vi "tapa color.vi"(9 "y":dbl=0.75, 10 "x":dbl=0.75, 11 "Image 2":T1) -> ()   [LabVIEW 2020]
uses:
  <vilib>/vision/Image Controls.llb/IMAQ Image.ctl
  <vilib>/vision/NI_Vision_Development_Module.lvlib
panel:
  out "Image":T1(plugin-control)
  in  "Color Sensitivity":u32(ring) items=["Low", "Medium", "High"]
  out "K":bool
  out "Color Spectrum":dbl[](array[numeric]) format="%.2f"
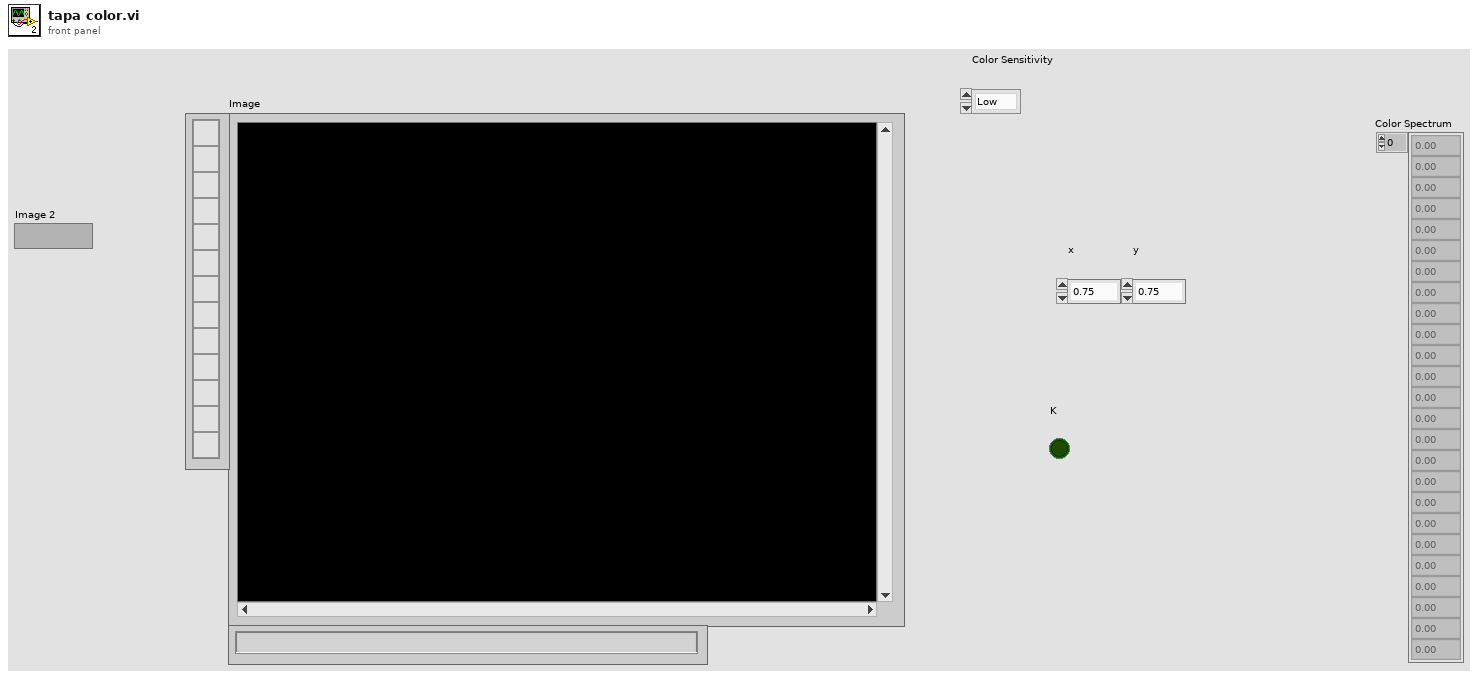
[diagram p1: front panel]
types:
  T1 = typedef "IMAQ Image.ctl" = refnum<image>
  T2 = cluster{"Global Rectangle":i32[], "Contours":cluster{"Contour Type":u32, "ROI Type":u32, "Points":i32[]}[]}
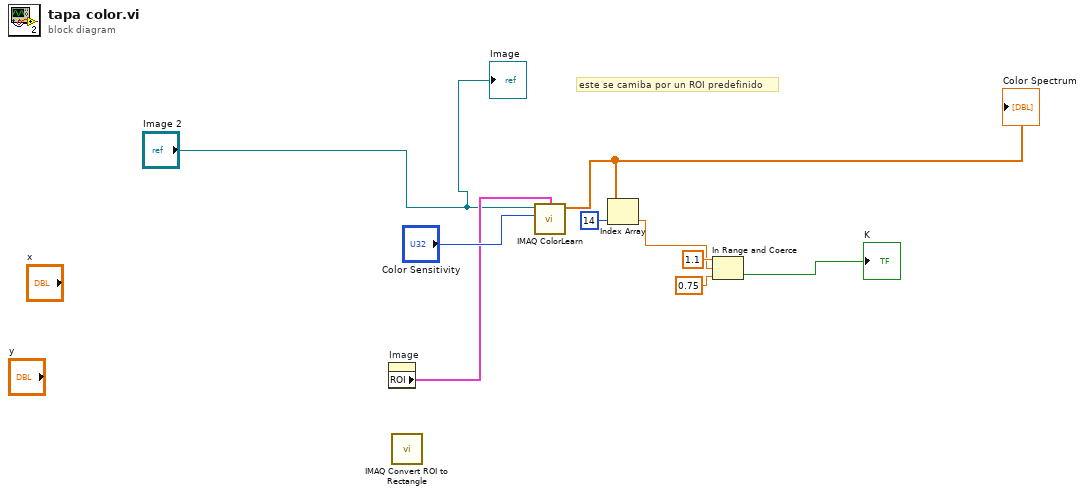
[diagram p0: block diagram]
diagram:
  # "este se camiba por un ROI predefinido"
  n1 = property on="Image" class="ImageControl"() -> ("ROI"=w3:T2)  [unwired: 2 in, 2 out]
  n2 = call "IMAQ Convert ROI to Rectangle"() -> ()  [unwired: 9 in, 2 out]
  n3 = call "IMAQ ColorLearn"("ROI Descriptor"=w3, "Image"="Image 2", "Color Sensitivity"="Color Sensitivity") -> ("Color Spectrum"=w8:dbl[])  [unwired: 5 in, 1 out]
  "Color Spectrum" <- w8
  n4 = Index Array(array=w8, index=14) -> (element=w1:dbl)
  n5 = In Range and Coerce(upper limit=1.1, x=w1, lower limit=0.75) -> (In Range?=→"K":bool)  [unwired: 1 out]
  "Image" <- "Image 2"
